vi "VARIABLE GLOBAL  GALGAS.vi"() -> ()   [LabVIEW 2015]
panel:
  out "PROMEDIO GALGAS":dbl
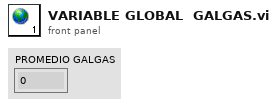
[diagram p1: front panel]
diagram:
